vi "Count Module Usage in Aliases.vi"(8 "error in (no error)":errorcluster, 10 "Module path":string, 11 "Alias Mappings":T1[](array[typedef])) -> (0 "error out":errorcluster, 3 "Number of Usages":i32)   [LabVIEW 2017, in "Routing and Faulting System Explorer.lvlib"]
uses:
  Routing and Faulting System Explorer.lvlib
  Shared/Alias Mapping.ctl
  Shared/Alias Endpoint.ctl
  Shared/Routing and Faulting Shared.lvlib
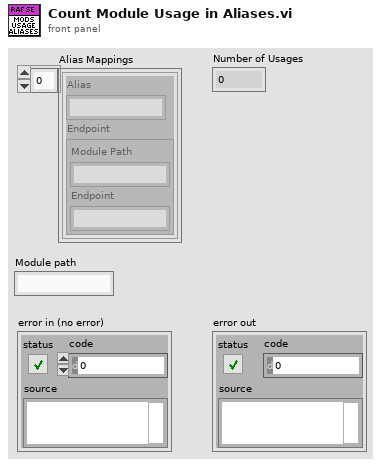
[diagram p1: front panel]
types:
  T1 = typedef "Routing and Faulting Shared.lvlib/Alias Mapping.ctl" = cluster{"Alias":string, "Endpoint":T2}
  T2 = typedef "Routing and Faulting Shared.lvlib/Alias Endpoint.ctl" = cluster{"Module Path":string, "Endpoint":string}
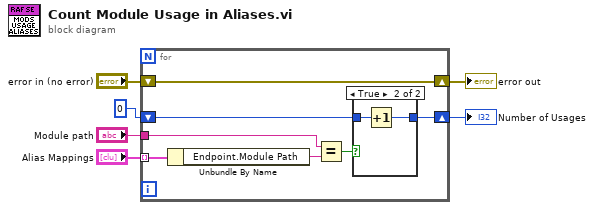
[diagram p0: block diagram]
diagram:
  n1 = for {
    tunnel: "Alias Mappings" -> [w11] mode=indexing
    shift-right: [w7] -> w3
    shift-left: "error in (no error)" -> [w7]
    tunnel: "Module path" -> [w13]
    shift-right: [w8] -> w6
    shift-left: 0 -> [w10]
    n2 = Unbundle By Name(w11) -> ("Endpoint.Module Path"=w12:string)
    n3 = Equal?(x=w13, y=w12) -> (x = y?=w9:bool)
    n4 = case shown="True" w9 {
      tunnel: w10 -> [w14 w16]
      tunnel: [w14 w15] -> w8
      frame False {
      }
      frame True {
        n5 = Increment(x=w16) -> (x+1=w15:i32)
      }
    }
  }
  "Number of Usages" <- w6
  "error out" <- w3
